vi "HTTP-GETRequest.vi"(6 "ResponseCode":string, 8 "error in (no error)":errorcluster, 9 "Parameter":string, 10 "Request":string, 11 "ByteGSWebAPI-V0 in":refnum<class "ByteGSWebAPI-V0.lvclass">) -> (0 "error out":errorcluster, 1 "Headers":string, 2 "Body":string, 3 "ByteGSWebAPI-V0 out":refnum<class "ByteGSWebAPI-V0.lvclass">)   [LabVIEW 2019, in "ByteGSWebAPI.lvlib" / "ByteGSWebAPI-V0.lvclass"]
doc: "Effettua una richiesta di GET al server come:\nSERVER/api/bytegs/RICHIESTA/PARAMETRO(opzionale)"
uses:
  ByteGSWebAPI-V0.lvclass
  ByteGSWebAPI-V0.lvclass/ByteGSWebAPI-V0.ctl
  <vilib>/httpClient/LabVIEWHTTPClient.lvlib
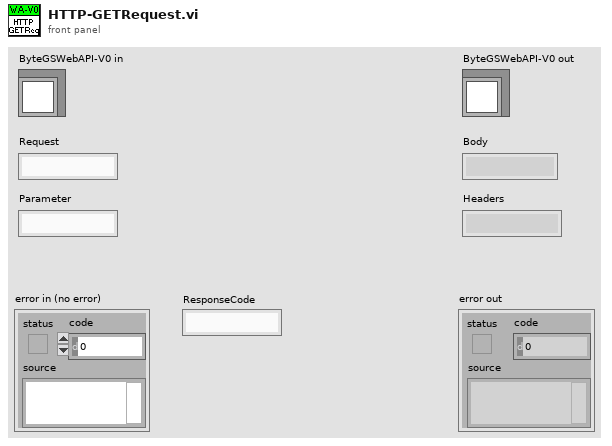
[diagram p1: front panel]
types:
  T1 = typedef "LabVIEWHTTPClient.lvlib/ClientHandle.ctl" = refnum<k1>
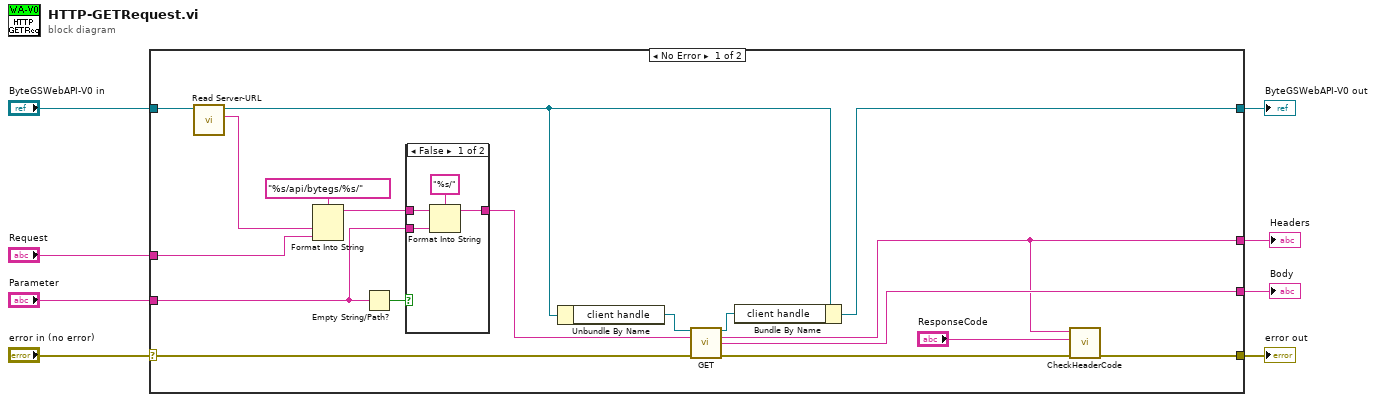
[diagram p0: block diagram]
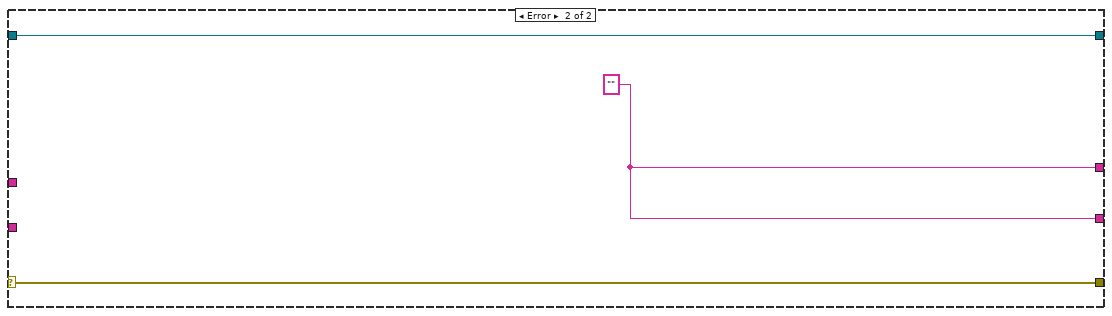
[diagram p3: hidden frame]
diagram:
  n1 = case shown="No Error" "error in (no error)" {
    selector: "error in (no error)" -> [w21 w34]
    tunnel: [w11 w34] -> w7
    tunnel: [w18 w33] -> w5
    tunnel: "ByteGSWebAPI-V0 in" -> [w13 w33]
    tunnel: "Request" -> [w23 _]
    tunnel: "Parameter" -> [w22 _]
    tunnel: [w17 w32] -> w2
    tunnel: [w9 w32] -> w1
    frame No Error {
      n2 = call-dynamic "Read Server-URL.vi"("ByteGSWebAPI-V0 in"=w13) -> ("Server-URL"=w15:string, "ByteGSWebAPI-V0 out"=w14:refnum<class "ByteGSWebAPI-V0.lvclass">)  [unwired: 8 in, 1 out]
      n3 = Format Into String(format string="%s/api/bytegs/%s/" ("url"), w15, w23) -> (resulting string=w25:string)  [unwired: 2 in, 1 out]
      n4 = Empty String/Path?(string/path=w22) -> (empty?=w24:bool)
      n5 = case shown="False" w24 {
        tunnel: w25 -> [w29 w31]
        tunnel: [w27 w31] -> w20
        tunnel: w22 -> [w28 _]
        frame False {
          n6 = Format Into String(format string="%s/" ("url"), initial string=w29, w28) -> (resulting string=w27:string)  [unwired: 1 in, 1 out]
        }
        frame True {
        }
      }
      n7 = Unbundle By Name(w14) -> ("client handle"=w19:T1)
      n8 = call <vilib>:"GET.vi"("client handle"=w19, "url"=w20, "error in (no error)"=w21) -> ("client handle out"=w16:T1, "headers"=w9:string, "body"=w17:string, "error out"=w12:errorcluster)  [unwired: 9 in]
      n9 = Bundle By Name(cluster=w14, "client handle"=w16) -> (w18:refnum<class "ByteGSWebAPI-V0.lvclass">)
      n10 = call "CheckHeaderCode.vi"("error in"=w12, "Code"="ResponseCode", "Headers"=w9) -> ("error out"=w11:errorcluster)  [unwired: 8 in]
    }
    frame Error {
      w32 = "" ("body")
    }
  }
  "error out" <- w7
  "ByteGSWebAPI-V0 out" <- w5
  "Body" <- w2
  "Headers" <- w1
